vi "PID Test.vi"() -> ()   [LabVIEW 2016]
uses:
  <vilib>/addons/control/pid/pid.llb/PID (DBL).vi
  <vilib>/addons/control/pid/NI_PID_pid.lvlib
panel:
  out "dt (s)":dbl
  out "Output":dbl
  in  "dt (s)":dbl
  in  "Deriviative Time (Td, Min)":dbl
  in  "Integral Time (Ti, min)":dbl
  in  "Proportional Gain (Kc)":dbl
  in  "Process Variable":dbl
  in  "Setpoint":dbl
  in  "Min Output":dbl
  in  "Max Output":dbl
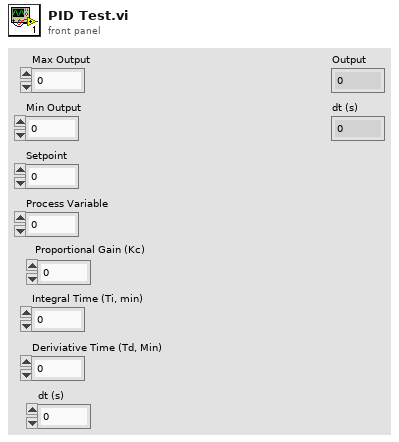
[diagram p1: front panel]
types:
  T1 = cluster{"Proportional Gain (Kc)":dbl, "Integral Time (Ti, min)":dbl, "Deriviative Time (Td, Min)":dbl}
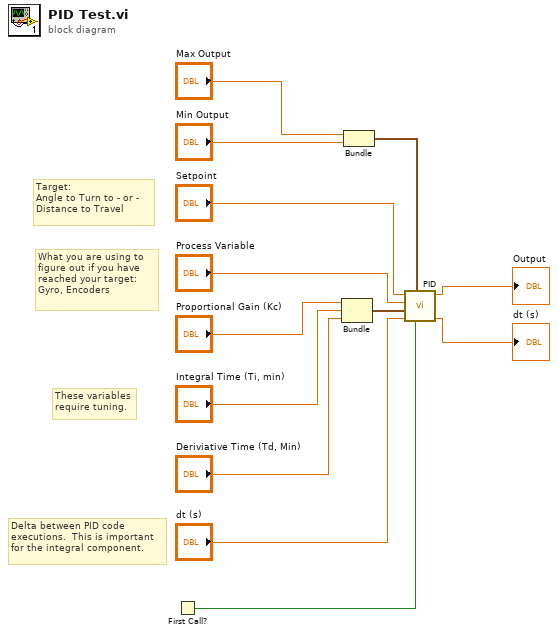
[diagram p0: block diagram]
diagram:
  # "Delta between PID code\nexecutions.  This is important\nfor the integral component."
  # "These variables\nrequire tuning."
  # "What you are using to \nfigure out if you have\nreached your target:\nGyro, Encoders"
  # "Target:\nAngle to Turn to - or -\nDistance to Travel"
  n1 = First Call?() -> (First Call?: T/F=w3:bool)
  n2 = Bundle("Proportional Gain (Kc)"="Proportional Gain (Kc)", "Integral Time (Ti, min)"="Integral Time (Ti, min)", "Deriviative Time (Td, Min)"="Deriviative Time (Td, Min)") -> (w5:T1)  [unwired: 1 in]
  n3 = Bundle("Max Output"="Max Output", "Min Output"="Min Output") -> (w11:cluster{"Max Output":dbl, "Min Output":dbl})  [unwired: 1 in]
  n4 = call-poly <vilib>:"PID.vi"("reinitialize? (F)"=w3, "output range"=w11, "dt (s)"="dt (s)", "PID gains"=w5, "process variable"="Process Variable", "setpoint"="Setpoint") -> ("dt out (s)"=→"dt (s)":dbl, "output"=→"Output":dbl)  [unwired: 4 in]
